vi "Update Digital Audio Generation (Freq and Amp).vi"(8 "error in":errorcluster, 9 "gain":dbl, 10 "frequency":dbl, 11 "Digital audio task":T1) -> (0 "error out":errorcluster, 3 "Digital audio task out":T1)   [LabVIEW 2021, in "Stepped Frequency Sweep_Audio DAC.lvlib"]
uses:
  <vilib>/PDM Acquisition Toolkit/host/Classes/Tasks/PCM Output/Controls/PCM Output Task DVR.ctl
  <vilib>/PDM Acquisition Toolkit/host/Classes/Tasks/PCM Output/PCM Output Task.lvclass
  C:/Program Files/National Instruments/LabVIEW 2021/vi.lib/PDM Acquisition Toolkit/host/Classes/Tasks/Parent/DecoderTask.lvclass
  <vilib>/PDM Acquisition Toolkit/host/Classes/Channels/PCM Output/PCM Output Channel.lvclass
  C:/Program Files/National Instruments/LabVIEW 2021/vi.lib/PDM Acquisition Toolkit/host/Classes/Channels/DecoderChannel.lvclass
  <vilib>/PDM Acquisition Toolkit/host/Classes/Channels/PCM Output/controls/PCM Output Channel - Signal Properties.ctl
  <vilib>/PDM Acquisition Toolkit/host/Classes/Channels/DecoderChannel.lvclass
  Stepped Frequency Sweep_Audio DAC.lvlib
  C:/Program Files/National Instruments/LabVIEW 2021/vi.lib/PDM Acquisition Toolkit/host/Classes/Channels/PCM Output/PCM Output Channel.lvclass
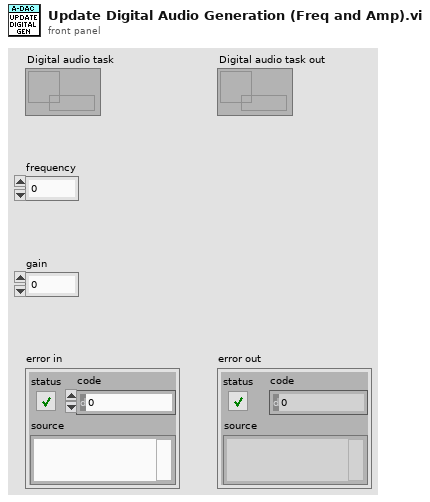
[diagram p1: front panel]
types:
  T1 = typedef "PDM Acquisition Class Library.lvlib/PCM Output Task.lvclass/PCM Output Task DVR.ctl" = refnum<data-value>
  T2 = typedef "PDM Acquisition Class Library.lvlib/PCM Output Channel.lvclass/PCM Output Channel - Signal Properties.ctl" = cluster{"cyclic period":dbl, "cyclic phase offset":dbl, "gain":dbl}
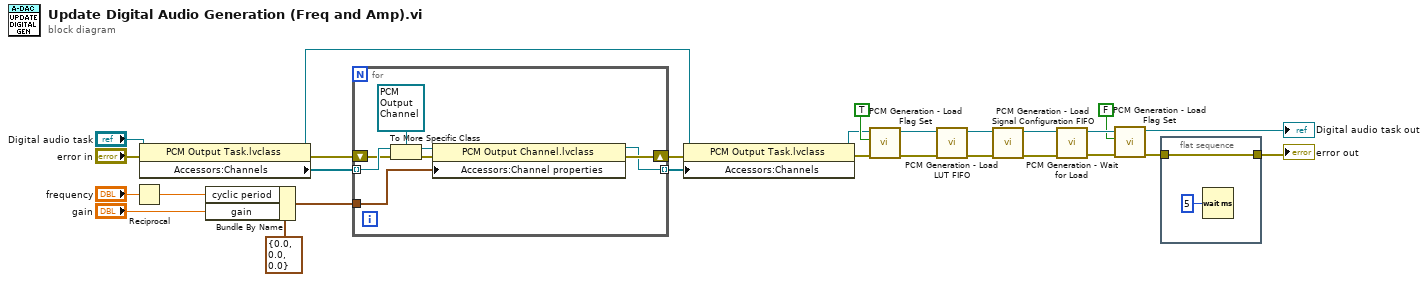
[diagram p0: block diagram]
diagram:
  n1 = Reciprocal(x="frequency") -> (1/x=w3:dbl)
  n2 = property class="PCM Output Task.lvclass"(reference="Digital audio task", error in="error in") -> (reference out=w14:T1, error out=w26:errorcluster, "Accessors:Channels"=w27:refnum<class "DecoderChannel.lvclass">[])
  n3 = Bundle By Name(cluster=T2 {"cyclic period"=0.0, "cyclic phase offset"=0.0, "gain"=0.0} ("Channel properties"), "cyclic period"=w3, "gain"="gain") -> (w1:T2)
  n4 = for {
    tunnel: w27 -> [w34] mode=indexing
    shift-right: [w30] -> w16
    shift-left: w26 -> [w32]
    tunnel: [w29] -> w15 mode=indexing
    tunnel: w1 -> [w28]
    n5 = To More Specific Class(target class=refnum<class "PCM Output Channel.lvclass"> refnum ("PDM Acquisition Class Library.lvlib:PCM Output Channel.lvclass"), reference=w34, error in=w32) -> (specific class reference=w31:refnum<class "PCM Output Channel.lvclass">, error out=w35:errorcluster)
    n6 = property class="PCM Output Channel.lvclass"(reference=w31, error in=w35, "Accessors:Channel properties"=w28) -> (reference out=w29:refnum<class "PCM Output Channel.lvclass">, error out=w30:errorcluster)
  }
  n7 = property class="PCM Output Task.lvclass"(reference=w14, error in=w16, "Accessors:Channels"=w15) -> (reference out=w13:T1, error out=w12:errorcluster)
  n8 = call <vilib>:"PCM Generation - Load Flag Set.vi"("error in"=w12, "Load"=TRUE, "PCM Output Task In"=w13) -> ("error out"=w20:errorcluster, "PCM Output Task Out"=w19:T1)  [unwired: 7 in]
  n9 = call <vilib>:"PCM Generation - Load LUT FIFO.vi"("error in"=w20, "PCM Output Task In"=w19) -> ("error out"=w17:errorcluster, "PCM Output Task Out"=w18:T1)  [unwired: 8 in]
  n10 = call <vilib>:"PCM Generation - Load Signal Configuration FIFO.vi"("error in"=w17, "PCM Output Task In"=w18) -> ("error out"=w11:errorcluster, "PCM Output Task Out"=w21:T1)  [unwired: 8 in]
  n11 = call <vilib>:"PCM Generation - Wait for Load.vi"("error in"=w11, "PCM Output Task In"=w21) -> ("error out"=w23:errorcluster, "PCM Output Task Out"=w24:T1)  [unwired: 7 in, 1 out]
  n12 = call <vilib>:"PCM Generation - Load Flag Set.vi"("error in"=w23, "Load"=FALSE, "PCM Output Task In"=w24) -> ("error out"=w8:errorcluster, "PCM Output Task Out"=→"Digital audio task out":T1)  [unwired: 7 in]
  n13 = flat-sequence {
    tunnel: w8 -> [w37]
    tunnel: [w37] -> w7
    frame #0 {
      n14 = Wait (ms)(milliseconds to wait=u32 5) -> ()  [unwired: 1 out]
    }
  }
  "error out" <- w7
